vi "Parse.vi"(8 "Error In":errorcluster, 9 "Tokens":refnum<class "Token.lvclass">[](array[class]), 11 "Compiler In":refnum<class "Compiler.lvclass">) -> (0 "Error Out":errorcluster, 1 "Abstract Syntax Tree":refnum<class "Root.lvclass">, 3 "Compiler Out":refnum<class "Compiler.lvclass">)   [LabVIEW 2018, in "Toolkit.lvlib" / "Compiler.lvclass"]
uses:
  Compiler.lvclass
  Nodes/Root/Root.lvclass
  Tokens/Token/Token.lvclass
  Compiler.lvclass/Compiler.ctl
  Parser/Parser.lvclass
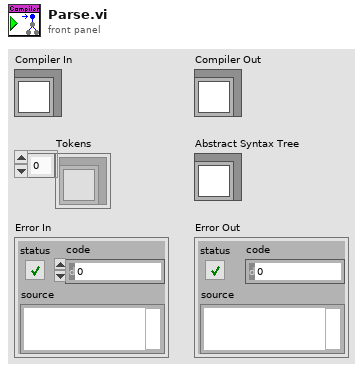
[diagram p1: front panel]
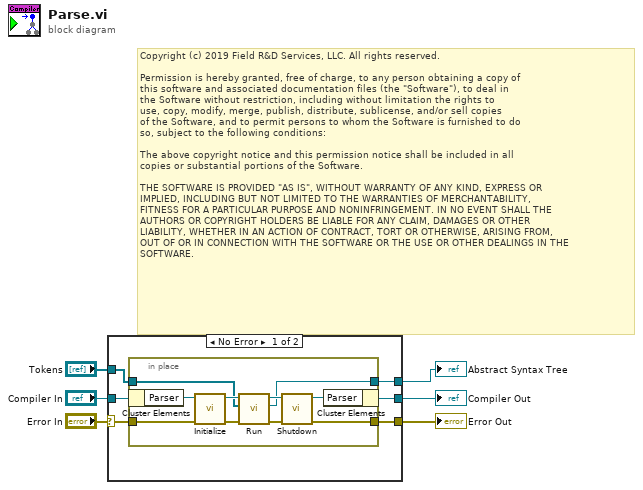
[diagram p0: block diagram]
diagram:
  # "Copyright (c) 2019 Field R&D Services, LLC. All rights reserved.\n\nPermission is hereby granted, free of charge, to any person obtaining a copy of\nthis software and associated documentation files (the \"Software\"), to deal in\nthe Software without restriction, including without limitation the rights to\nuse, copy, modify, merge, publish, distribute, sublicense, and/or sell copies\nof the Software, and to permit persons to whom the Software is furnished to do\nso, subject to the following conditions:\n\nThe above copyright notice and this permission notice shall be included in all\ncopies or substantial portions of the Software.\n\nTHE SOFTWARE IS PROVIDED \"AS IS\", WITHOUT WARRANTY OF ANY KIND, EXPRESS OR\nIMPLIED, INCLUDING BUT NOT LIMITED TO THE WARRANTIES OF MERCHANTABILITY,\nFITNESS FOR A PARTICULAR PURPOSE AND NONINFRINGEMENT. IN NO EVENT SHALL THE\nAUTHORS OR COPYRIGHT HOLDERS BE LIABLE FOR ANY CLAIM, DAMAGES OR OTHER\nLIABILITY, WHETHER IN AN ACTION OF CONTRACT, TORT OR OTHERWISE, ARISING FROM,\nOUT OF OR IN CONNECTION WITH THE SOFTWARE OR THE USE OR OTHER DEALINGS IN THE\nSOFTWARE."
  n1 = case shown="No Error" "Error In" {
    selector: "Error In" -> [w10 w24]
    tunnel: [w9 w24] -> w5
    tunnel: "Tokens" -> [w11 _]
    tunnel: "Compiler In" -> [w12 w23]
    tunnel: [w8 w23] -> w2
    tunnel: [w7 _] -> w1
    frame No Error {
      n2 = in-place {
        in-place-border: w11 -> [w19]
        in-place-border: w10 -> [w18]
        in-place-border: [w15] -> w9
        in-place-border: [w13] -> w7
        n3 = in-place-cluster #1(w12) -> ("Parser"=w22:refnum<class "Parser.lvclass">)
        n4 = call-dynamic "Initialize.vi"("Error In"=w18, "Parser In"=w22) -> ("Error Out"=w20:errorcluster, "Parser Out"=w21:refnum<class "Parser.lvclass">)  [unwired: 8 in]
        n5 = call-dynamic "Run.vi"("Error In"=w20, "Tokens"=w19, "Parser In"=w21) -> ("Error Out"=w16:errorcluster, "Abstract Syntax Tree"=w13:refnum<class "Root.lvclass">, "Parser Out"=w17:refnum<class "Parser.lvclass">)  [unwired: 6 in]
        n6 = call-dynamic "Shutdown.vi"("Error In"=w16, "Parser In"=w17) -> ("Error Out"=w15:errorcluster, "Parser Out"=w14:refnum<class "Parser.lvclass">)  [unwired: 8 in]
        n7 = in-place-cluster #1("Parser"=w14) -> (w8:refnum<class "Compiler.lvclass">)
      }
    }
    frame Error {
    }
  }
  "Error Out" <- w5
  "Abstract Syntax Tree" <- w1
  "Compiler Out" <- w2
